vi "GUI_kHz_FlexibleDelivery.vi"() -> ()   [LabVIEW 2020]
uses:
  Shared/GUI_Template/GUI_master/tcp_new_data_event.ctl
  Shared/GUI_Template/GUI_master/tcp new data cluster.ctl
panel:
  in  "BASE PATH":path=path "Z:/software/control-all-loasis/kHzLPA/Active Version"
  in  "stop":bool=TRUE
  in  "Tab Control":T1(tab)=enum."Experts Only"
  in  "GUIdevice 19":string="kHz_Cam2-3_AstrellaMode"
  in  "GUIdevice 14":string="KHz_Cam68-1_ghost"
  in  "GUIdevice 13":string="kHz_Cam1-4_Astrella-Spol"
  in  "GUIdevice 6":string="kHz_Pico8742_EC"
  in  "GUIdevice 2":string="kHz_1Wire"
  in  "GUIdevice 1":string="kHz_ManualParameter"
  in  "GUIdevice 3":string="kHz_Zaber_Vacuum"
  in  "GUIdevice 4":string="kHz_DG645_ShotControl"
  in  "GUIdevice 5":string="kHz_Pico8742_CC"
  out "error IO":errorcluster
  out "tcp data event":T2
  in  "GUIdevice 7":string="kHz_ESP_TC"
  in  "GUIdevice 8":string="kHz_Pico8742_GLO"
  in  "GUIdevice 9":string="kHz_Pico8742_ROT"
  in  "GUIdevice 10":string="kHz_FilterWheel_splitter"
  in  "GUIdevice 11":string="kHz_Cam42-4_NFProfileOL"
  in  "GUIdevice 12":string="kHz_Cam42-2_EC"
  in  "GUIdevice 15":string="kHz_Cam42-2_EC"
  in  "GUIdevice 16":string="kHz_Cam42-4_NFProfileOL"
  in  "GUIdevice 18":string="kHz_Cam68-3_MantaG-158"
  in  "GUIdevice 17":string="kHz_Cam68-2_SpolGhost"
  in  "Position.Channel 1::2":T3(ring) caption="Mode Flipper"
  in  "step size EC":i32=200 caption="Step Size" min=10 max=1000 step=10
  in  "step size GLO":i32=200 caption="Step Size" min=10 max=1000 step=10
  in  "step size CC":i32=200 caption="Step Size" min=10 max=1000 step=10
  in  "value8::1":i8=-3 caption="Round Trip" min=-4 max=0 step=1 format="%.0g"
  in  "value7::1":dbl=35.0 caption="HWP attenuator" min=-9999999.0 max=9999999.0
  out "HCF output energy":dbl=7.782297644090318 caption="HCF output energy [uJ]"
  in  "Position.device 3::6":i32=450 caption="EC H" min=-1000 max=1000 step=200
  in  "Position.device 4::6":i32=1350 caption="EC V" min=-1000 max=1000 step=200
  in  "Position.device 1::5":i32=-8149 caption="Near H" min=-20000 max=20000 step=50
  in  "Position.device 2::5":i32=-10850 caption="Near V" min=-20000 max=20000 step=50
  in  "Position.device 1::8":i32=100 caption="Far V" min=-100000 max=100000 step=200
  in  "Position.device 2::8":i32=-69835 caption="Far H" min=-100000 max=100000 step=200
  in  "Position.device 3::8":i32=-48990 caption="OAP V" min=-100000 max=100000 step=200
  in  "Position.device 4::8":i32=12420 caption="OAP H" min=-100000 max=100000 step=200
  in  "p-pol only button":bool=TRUE caption="p-pol only"
  in  "Position.Axis 3::7":dbl=23.00005 caption="Mode Wedge Position" min=0.0 max=25.0 format="%.2f"
  in  "Position.Ch2::3":dbl=53.000052 caption="Manta Cam Position" min=0.0 max=100.0 format="%.2f"
  in  "Mode Wedge Button":bool=TRUE caption="Mode Wedge In"
  in  "UDP error message":string
  out "Attenuated  Power":dbl=11.11756806298617 caption="Attenuated Power [mW]"
  out "FF input calculated":dbl=1.5564595288180636 caption="FF input  [uJ]"
  out "FF input OL":dbl=-2.9732313575525815 caption="FF input OL s+p [mW]"
  out "chart":cluster{"energy":dbl, "energy":dbl, dbl}(graph)={"energy"=-2.9732313575525815, "energy"=-2.9732313575525815, 100.0}
  out "FF Output OL":dbl=-2.9732313575525815 caption="FF output OL  [uJ]"
  in  "value10::1":dbl=0.017 caption="FF input slope" min=-9999999.0 max=9999999.0
  in  "value12::1":dbl=52.3 caption="FF Output Divisor" min=-9999999.0 max=9999999.0
  in  "MeanCounts::16":dbl caption="NFProfileOL Mean" min=0.0 max=999999999.0 format="%.2f"
  in  "pos.Channel0::10":enum16{"1", "2", "3", "4", "5", "6"}(ring)=enum."6" caption="Filter Wheel"
  in  "value5::1":dbl caption="HWP splitter" min=-9999999.0 max=9999999.0
  in  "Astrella Power":dbl[](array[numeric])=[5470.0, 3400.0, 690.0, 135.0, 20.0] caption="Astrella Power [mW]"
  in  "value1::1":dbl=21.7 caption="Revo current" min=10.0 max=30.0
  in  "exposure::16":dbl=0.001 caption="NFProfileOL exposure" min=1e-05 max=1.0 format="%.2f"
  in  "Position.device 1::9":i32=10000 caption="WP in CC" min=-10000 max=10000 step=200
  in  "step size ROT":i32=200 caption="Step Size" min=10 max=1000 step=10
  in  "MeanCounts::12":dbl caption="EC Mean" min=0.0 max=999999999.0 format="%.2f"
  in  "exposure::12":dbl=0.001 caption="EC exposure" min=1e-05 max=10.0 format="%.2f"
  in  "Max Exposure - Ghost":dbl=0.25
  in  "Max Exposure - Astrellas":dbl=0.25
  in  "GuardBand Ghost":dbl=20.0
  in  "Guardband Astrellas":dbl=100.0
  in  "Target - Ghost":dbl=170.0
  in  "Target - Astrellas":dbl=3000.0
  in  "Exposure Step Size - Ghost":dbl=0.02
  in  "Exposure Step Size - Astrellas":dbl=0.02
  in  "exposure::13":dbl=23.00005 caption="Exposure - Astrellas" min=1e-05 max=10.0 format="%.4f"
  in  "exposure::14":dbl=23.00005 caption="Exposure - Ghost" min=1e-05 max=1.0 format="%.4f"
  in  "maxcounts::13":dbl=23.00005 caption="MaxCounts - Astrellas" min=0.0 max=999999999.0 format="%.2f"
  in  "maxcounts::14":dbl=23.00005 caption="MaxCounts - Ghost" min=0.0 max=999999999.0 format="%.2f"
  in  "On":bool caption="Auto Exposure"
  out "timer":u32
  in  "Exposure Step Size -EC":dbl=0.02
  in  "Target - EC":dbl=3000.0
  in  "Max Exposure -EC":dbl=0.5
  in  "GuardBand - EC":dbl=200.0
  in  "Exposure Step Size -NFProfile":dbl=0.02
  in  "Max Exposure - NFProfile":dbl=1.0
  in  "GuardBand - NFProfile":dbl=200.0
  in  "Target -  NFProfile":dbl=3000.0
  in  "Max Exposure - SpolGhost":dbl=0.5
  in  "Exposure Step Size - SpolGhost":dbl=0.02
  in  "GuardBand - SpolGhost":dbl=200.0
  in  "Target - SpolGhost":dbl=3000.0
  in  "Max Exposure - MantaG":dbl=0.5
  in  "Exposure Step Size - MantaG":dbl=0.02
  in  "GuardBand - MantaG":dbl=200.0
  in  "Target -  MantaG":dbl=3000.0
  in  "Target -  AstrellaM":dbl
  in  "GuardBand - AstrellaM":dbl
  in  "Exposure Step Size - AstrellaM":dbl=0.02
  in  "Max Exposure - AstrellaM":dbl=1.0
  in  "maxcounts::16":dbl=23.00005 caption="MaxCounts - NFProfile" min=0.0 max=999999999.0 format="%.2f"
  in  "exposure::16":dbl=23.00005 caption="Exposure - NFProfile" min=1e-05 max=1.0 format="%.4f"
  in  "exposure::17":dbl=23.00005 caption="Exposure - SPol" min=1e-05 max=1.0 format="%.4f"
  in  "maxcounts::17":dbl=23.00005 caption="MaxCounts - SPol" min=0.0 max=999999999.0 format="%.2f"
  in  "maxcounts::18":dbl=23.00005 caption="MaxCounts - Manta" min=0.0 max=999999999.0 format="%.2f"
  in  "exposure::18":dbl=23.00005 caption="Exposure - Manta" min=1e-05 max=1.0 format="%.4f"
  in  "exposure::19":dbl=23.00005 caption="Exposure - AstrellaM" min=1e-05 max=1.0 format="%.4f"
  in  "maxcounts::19":dbl=23.00005 caption="MaxCounts - AstrellaM" min=0.0 max=999999999.0 format="%.2f"
  in  "exposure::15":dbl=23.00005 caption="Exposure - EC" min=1e-05 max=10.0 format="%.4f"
  in  "maxcounts::15":dbl=23.00005 caption="MaxCounts - EC" min=0.0 max=999999999.0 format="%.2f"
  # "Flexible Delivery"
  # "Primary Controls"
  # "Laser Status"
  # "OL Measurement"
  # "Calculated"
  # "Alignment Near-field"
  # "EC focus tuning"
  # "Beam centering on in-flange Gentec"
  # "DON'T TOUCH"
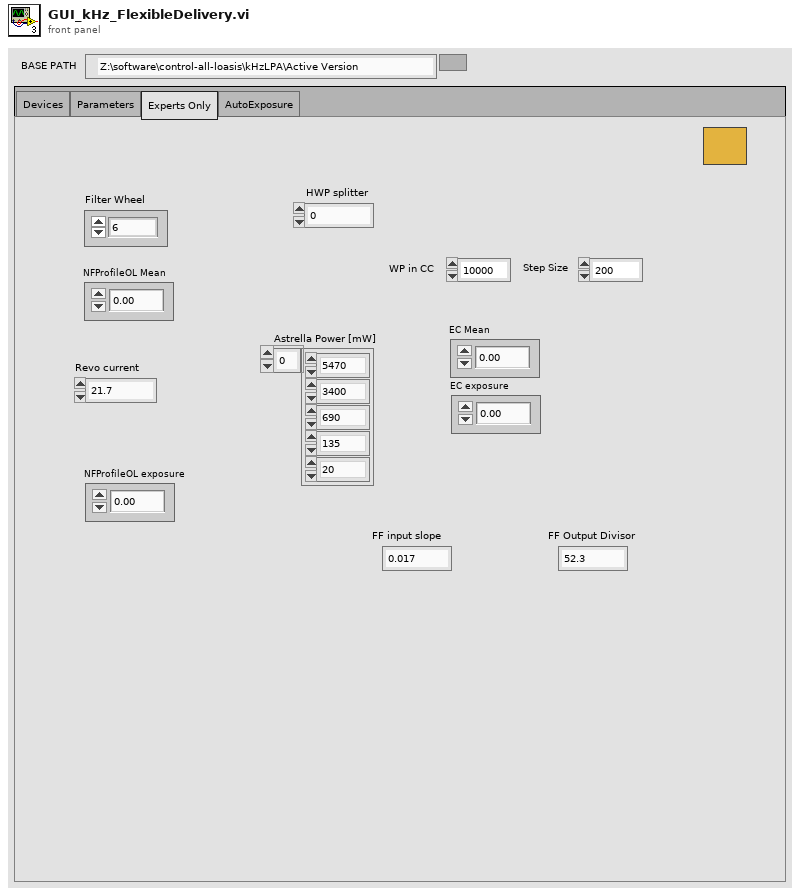
[diagram p1: front panel]
types:
  T1 = enum32{"Devices", "Parameters", "Experts Only", "AutoExposure"}
  T2 = typedef "tcp_new_data_event.ctl" = refnum<user-event>
  T3 = enum16{"Removed", "Inserted", "Unknown", "Moving"}
  T4 = typedef "tcp new data cluster.ctl" = cluster{"EventEnum":enum16{"new data", "connection status update"}, "Device name":string}
  T5 = enum32{"Invalid", "Standard", "Closed", "Hidden", "Minimized", "Maximized"}
  T6 = enum32{"invalid app kind", "Development System", "Run Time System", "Student Edition", "Embedded LabVIEW", "Evaluation", "Custom"}
  T7 = cluster{"Core":cluster{"Current VI Reference":refnum<vi>, "Close Panel on Exit?":bool}, "Tik1":u32}
  T8 = cluster{"Current VI Reference":refnum<vi>, "Close Panel on Exit?":bool}
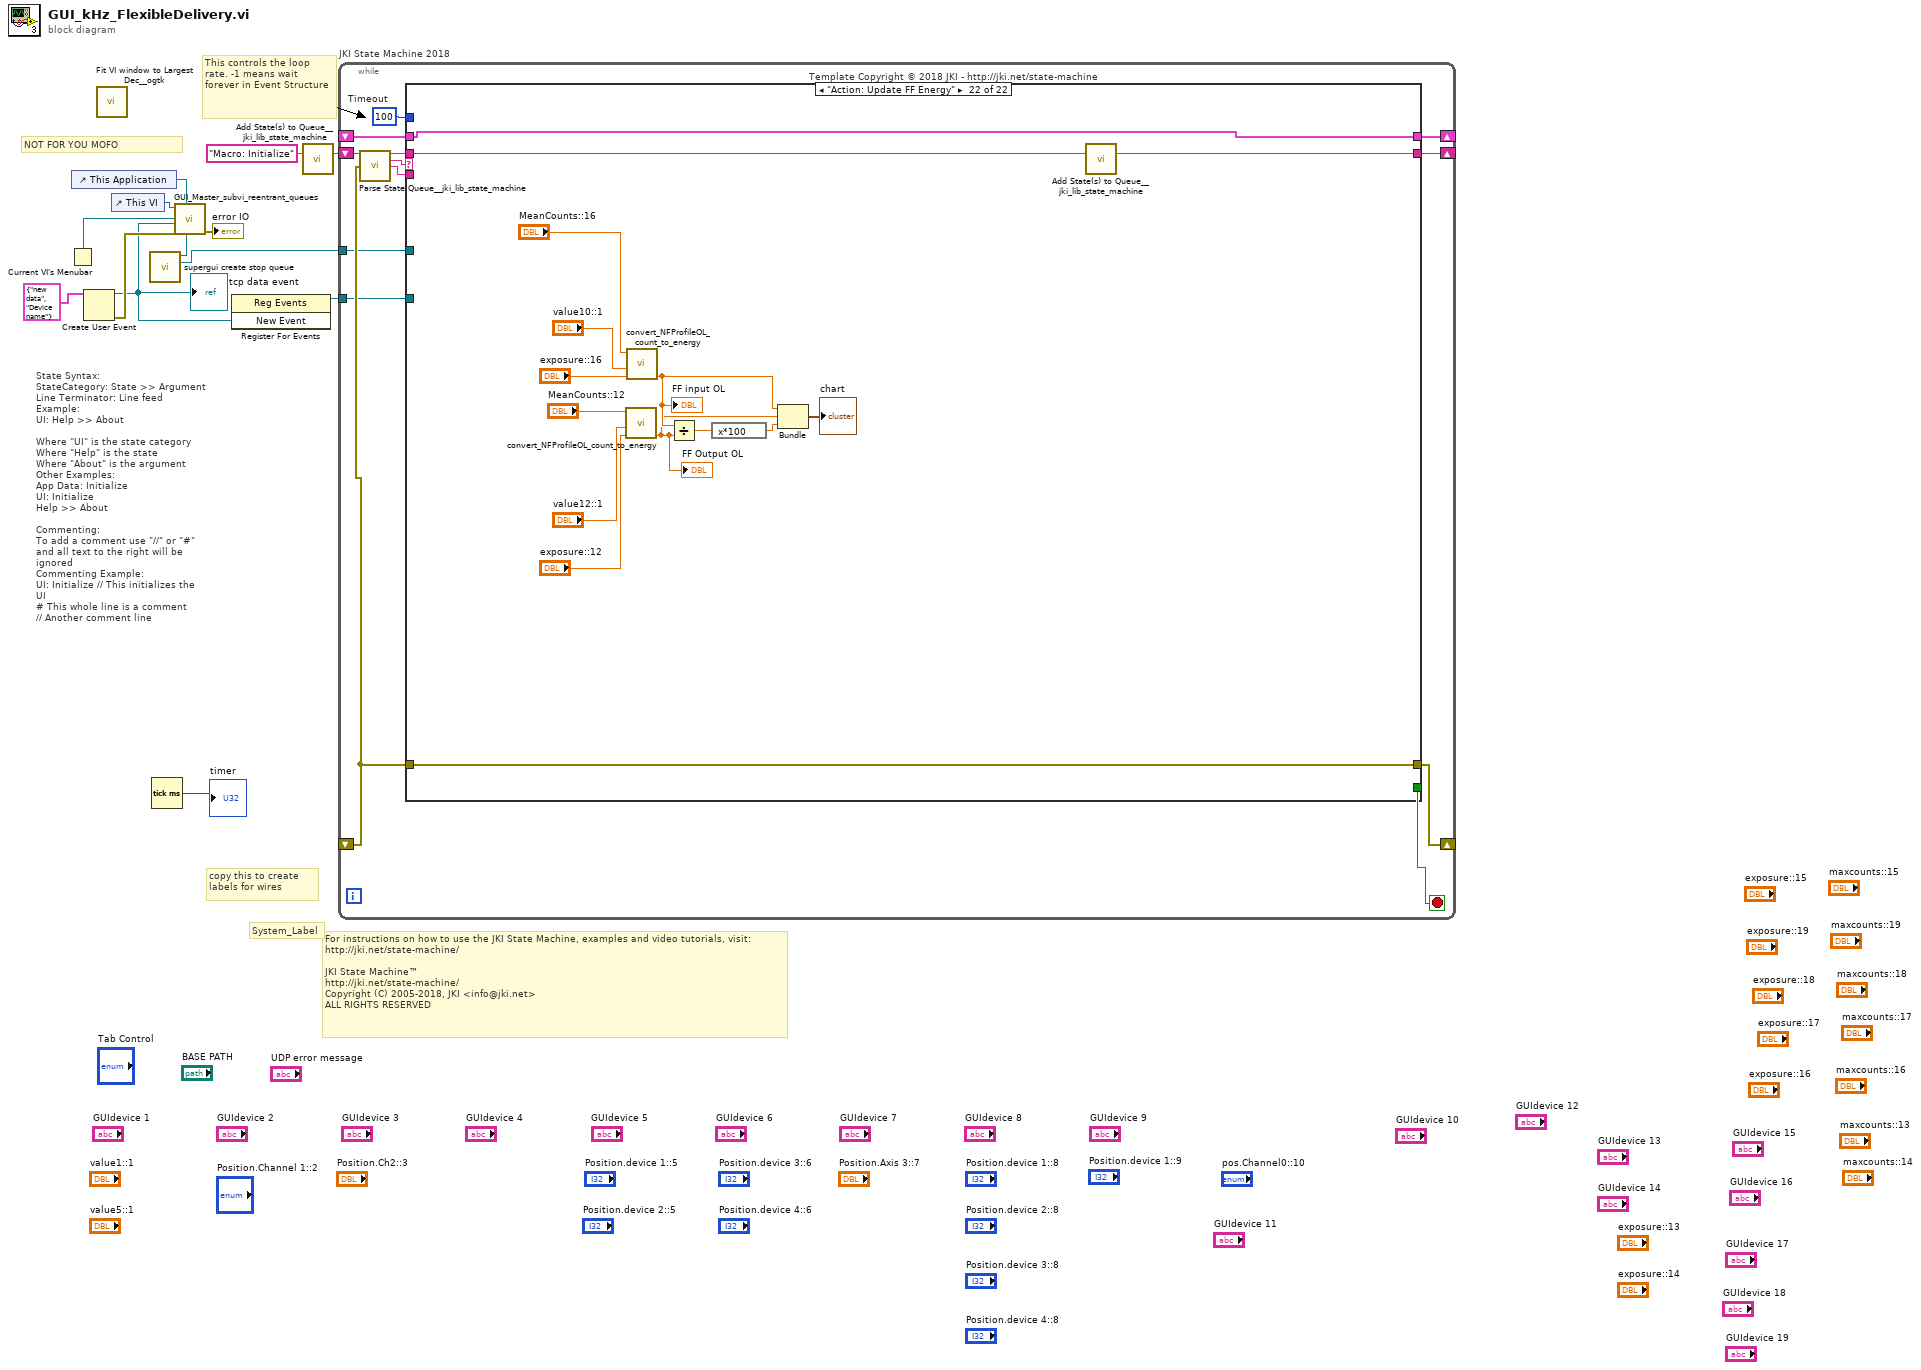
[diagram p0: block diagram]
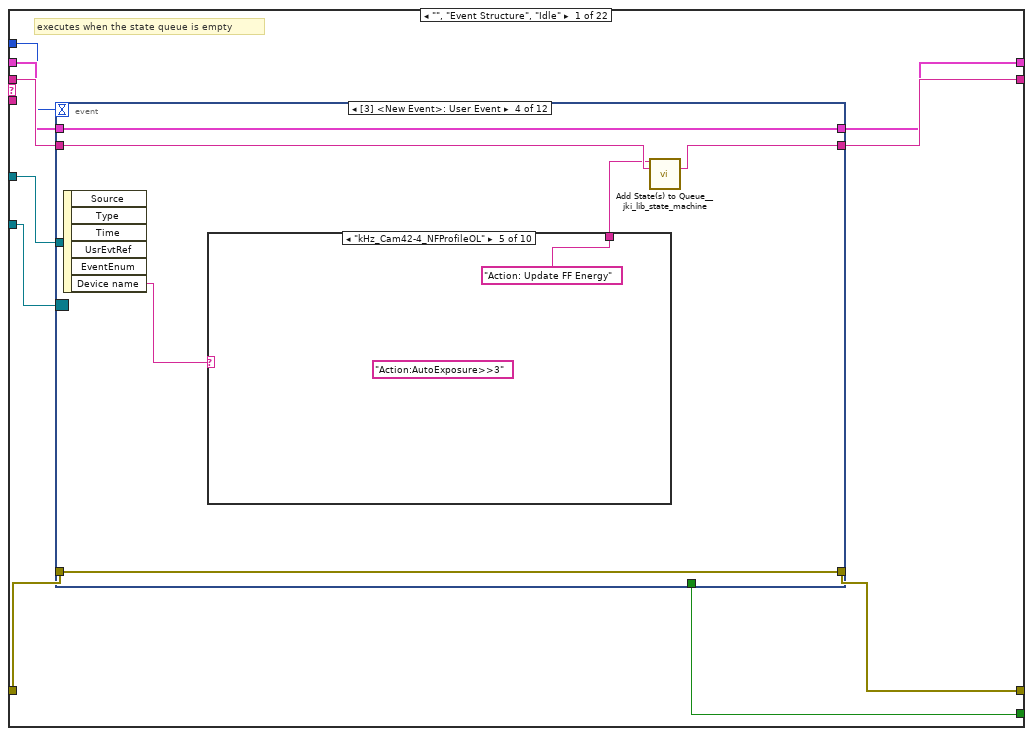
[diagram p2: hidden frame]
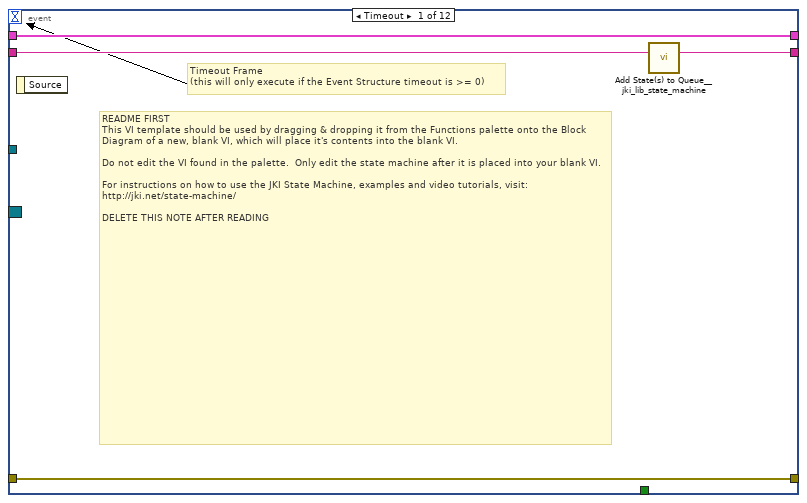
[diagram p3: hidden frame]
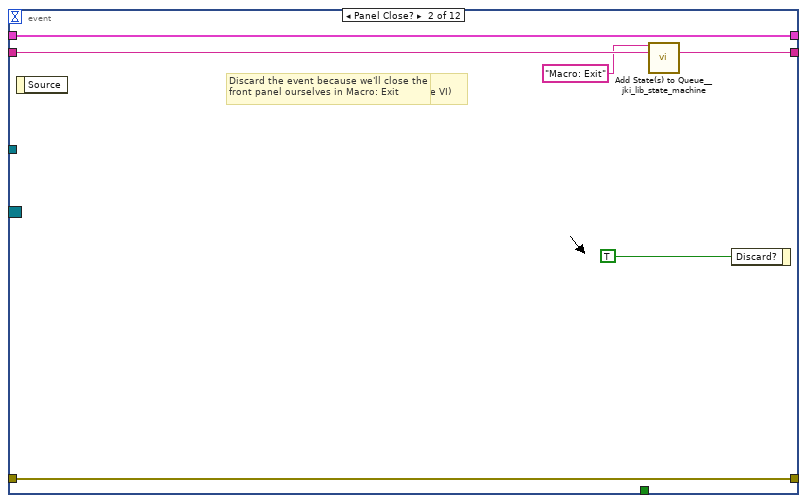
[diagram p4: hidden frame]
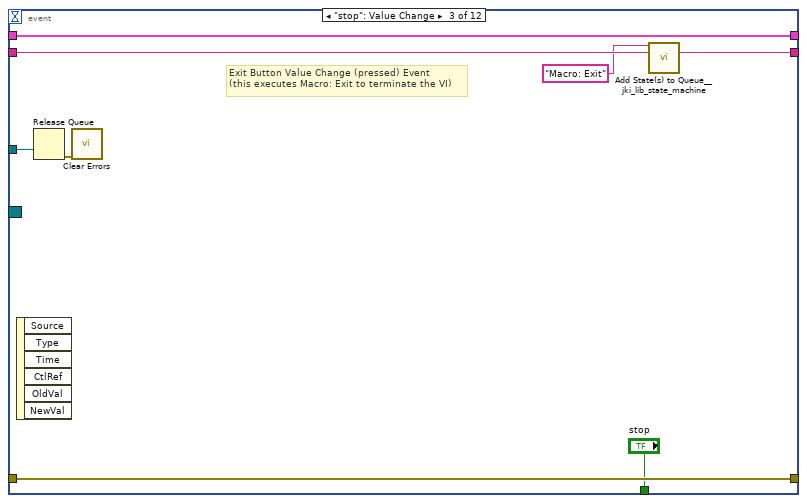
[diagram p5: hidden frame]
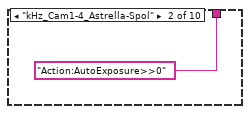
[diagram p7: hidden frame]
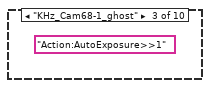
[diagram p8: hidden frame]
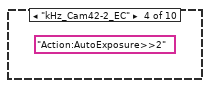
[diagram p9: hidden frame]
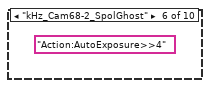
[diagram p10: hidden frame]
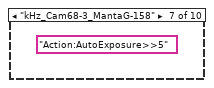
[diagram p11: hidden frame]
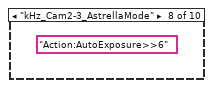
[diagram p12: hidden frame]
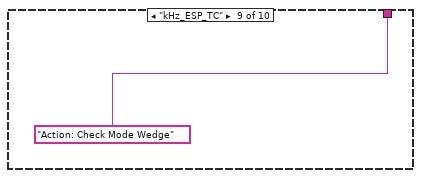
[diagram p13: hidden frame]
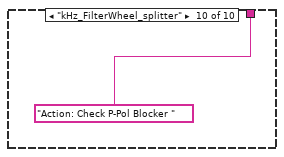
[diagram p14: hidden frame]
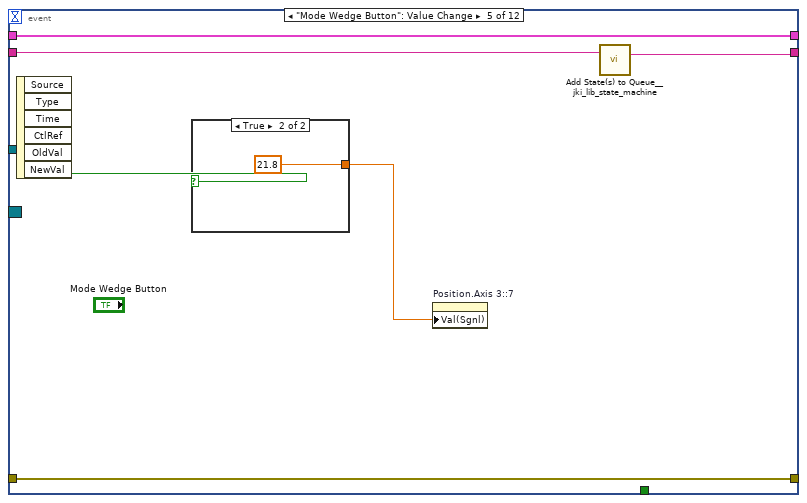
[diagram p15: hidden frame]
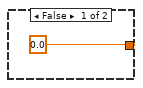
[diagram p16: hidden frame]
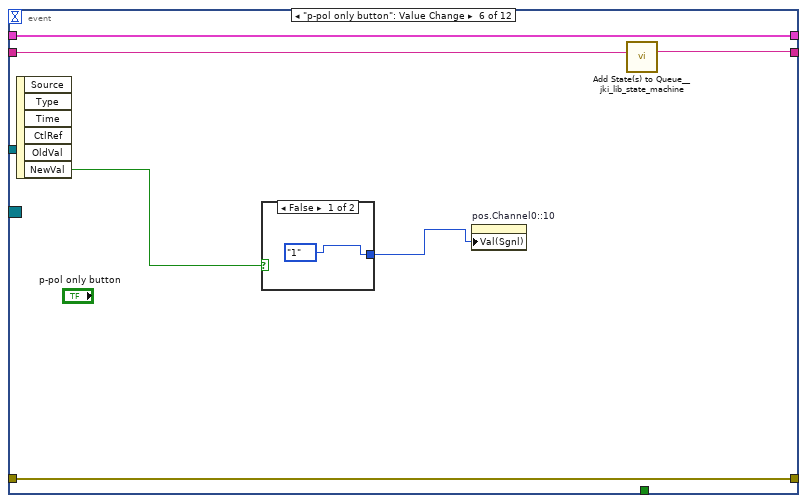
[diagram p17: hidden frame]
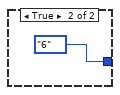
[diagram p18: hidden frame]
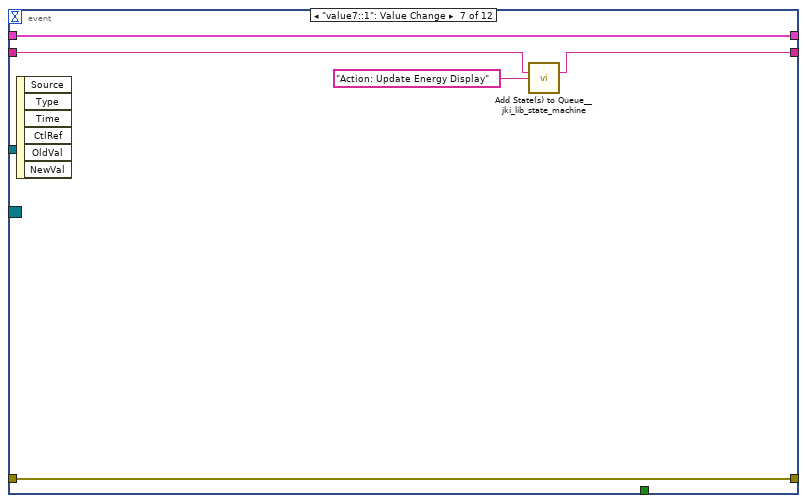
[diagram p19: hidden frame]
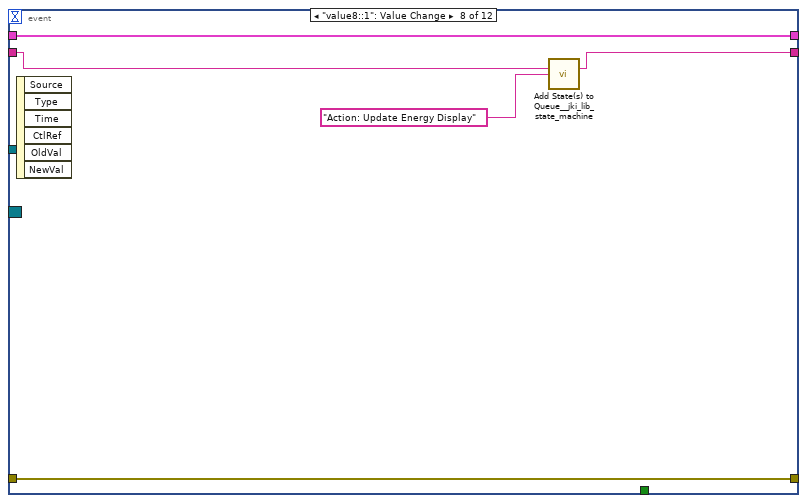
[diagram p20: hidden frame]
diagram:
  # "NOT FOR YOU MOFO"
  # "For instructions on how to use the JKI State Machine, examples and video tutorials, visit:\nhttp://jki.net/state-machine/\n\nJKI State Machine™\nhttp://jki.net/state-machine/\nCopyright (C) 2005-2018, JKI <info@jki.net>\nALL RIGHTS RESERVED"
  # "State Syntax:\nStateCategory: State >> Argument\nLine Terminator: Line feed\nExample:\nUI: Help >> About\n\nWhere \"UI\" is the state category\nWhere \"Help\" is the state\nWhere \"About\" is the argument\nOther Examples:\nApp Data: Initialize\nUI: Initialize\nHelp >> About\n\nCommenting:\nTo add a comment use \"//\" or \"#\" and all text to the right will be ignored\nCommenting Example:\nUI: Initialize // This initializes the UI\n# This whole line is a comment\n// Another comment line"
  # "copy this to create labels for wires"
  # "This controls the loop rate. -1 means wait forever in Event Structure"
  # "System_Label"
  n1 = Current VI's Menubar() -> (w7:refnum<k9>)
  n2 = control-ref of="This Application"() -> (w10:refnum<vi>)
  n3 = Create User Event(user event datatype=T4 {"EventEnum"=enum."new data", "Device name"="Device name"} ("New Event")) -> (user event=w4:refnum<user-event>, error out=w9:errorcluster)  [unwired: 1 in]
  "tcp data event" <- w4
  n4 = call <userlib>:"Fit VI window to Largest Dec__ogtk.vi"() -> ()  [unwired: 6 in, 2 out]
  n5 = control-ref of="This VI"() -> (w6:refnum<vi>)
  n6 = call "supergui create stop queue.vi"() -> ("STOP Queue out"=w3:refnum<queue>)  [unwired: 11 in]
  n7 = Tick Count (ms)() -> (millisecond timer value=→"timer":u32)
  n8 = call "GUI_Master_subvi_reentrant_queues.vi"("STOP Queue in"=w3, "This Application"=w10, "error in (no error)"=w9, "tcp data event"=w4, "Caller menu reference"=w7, "Caller VI ref"=w6) -> ("error out"=→"error IO":errorcluster)  [unwired: 5 in]
  n9 = register-events(w4) -> (reference out=w2:refnum<event-registration>)  [unwired: 2 in, 1 out]
  n10 = call <vilib>:"Add State(s) to Queue__jki_lib_state_machine.vi"("State(s) in (\"\")"="Macro: Initialize") -> ("States Out"=w12:string)  [unwired: 14 in]
  n11 = while "JKI State Machine 2018" {
    shift-right: [w18] -> _
    shift-left: _ -> [w17]
    shift-right: [w21] -> _
    shift-left: _ -> [w15]
    shift-right: [w20] -> _
    shift-left: w12 -> [w22]
    tunnel: w3 -> [w14]
    tunnel: w2 -> [w13]
    stop <- w19 stop-if-true
    w16 = 100  # Timeout
    # "Template Copyright © 2018 JKI - http://jki.net/state-machine"
    n12 = call <vilib>:"Parse State Queue__jki_lib_state_machine.vi"("State Queue"=w22, "Error In (no error)"=w15) -> ("Remaining States"=w24:string, "Current State"=w25:string, "Arguments"=w23:string)  [unwired: 11 in]
    n13 = case shown="\"Action: Update FF Energy\"" w25 {
      selector: w25 -> [_ _ w114 _ _ _ _ _ _ _ _ _ _ _ _ _ _ _ _ _ _ _]
      tunnel: w24 -> [w35 w113 w118 w137 w143 w148 w152 w159 w165 w169 w173 w179 w190 w254 w259 w269 w273 w284 w437 w444 w454 w469]
      tunnel: w23 -> [_ _ _ _ _ _ _ _ _ _ _ w174 w184 _ _ _ _ w276 _ _ _ _]
      tunnel: w17 -> [w33 w110 w116 w130 w140 w146 w149 w153 w161 w166 w171 w177 w186 w251 w256 w266 w270 w281 w429 w438 w451 w466]
      tunnel: [w32 w111 w120 w134 errorcluster {"status"=FALSE, "code"=0, "source"=""} ("error out") w145 w150 w157 w162 w167 w170 w175 w187 w252 w257 w267 w271 w282 w435 w442 w452 w467] -> w21
      tunnel: w15 -> [w31 w111 w119 w134 w139 w145 w150 w157 w163 w167 w170 w176 w188 w252 w257 w267 w271 w282 w435 w442 w452 w467]
      tunnel: [w34 w112 w117 w136 w142 w147 w151 w158 w164 w168 w172 w178 w189 w253 w258 w268 w272 w283 w436 w443 w453 w468] -> w20
      tunnel: [w27 _ _ _ _ TRUE _ _ _ _ _ _ _ _ _ _ _ _ _ _ _ _] -> w19
      tunnel: [w30 w110 w116 w135 w140 w146 w149 w154 w161 w166 w171 w177 w186 w251 w256 w266 w270 w281 w429 w438 w451 w466] -> w18
      tunnel: w16 -> [w29 _ _ _ _ _ _ _ _ _ _ _ _ _ _ _ _ _ _ _ _ _]
      tunnel: w14 -> [w28 _ _ _ _ _ _ _ _ _ _ _ _ _ _ _ _ _ _ _ _ _]
      tunnel: w13 -> [w26 _ _ _ _ _ _ _ _ _ _ _ _ _ _ _ _ _ _ _ _ _]
      frame "", "Event Structure", "Idle" {
        # "executes when the state queue is empty"
        n14 = event shown="[3] <New Event>: User Event" {
          selector: w26 -> [_ _ _ _ _ _ _ _ _ _ _ _]
          dyn-events: _ -> [_ _ _ _ _ _ _ _ _ _ _ _]
          timeout: w29 -> [_ _ _ _ _ _ _ _ _ _ _ _]
          tunnel: w35 -> [w39 w45 w53 w57 w68 w74 w84 w87 w94 w99 w104 w109]
          tunnel: [w38 w44 w52 w58 w69 w75 w83 w89 w93 w98 w103 w108] -> w34
          tunnel: w33 -> [w36 w42 w50 w59 w64 w72 w82 w88 w92 w97 w102 w107]
          tunnel: [w37 w43 w51 w54 w66 w76 w81 w86 w91 w96 w101 w106] -> w32
          tunnel: w31 -> [w37 w43 w51 w54 w66 w76 w81 w86 w91 w96 w101 w106]
          tunnel: [w36 w42 w50 w59 w64 w72 w82 w88 w92 w97 w102 w107] -> w30
          tunnel: w28 -> [_ _ w47 _ _ _ _ _ _ _ _ _]
          tunnel: [_ _ "stop" _ _ _ _ _ _ _ _ _] -> w27
          event Timeout {
            # "README FIRST\nThis VI template should be used by dragging & dropping it from the Functions palette onto the Block Diagram of a new, blank VI, which will place it's contents into the blank VI.\n\nDo not edit the VI found in the palette.  Only edit the state machine after it is placed into your blank VI.\n\nFor instructions on how to use the JKI State Machine, examples and video tutorials, visit:\nhttp://jki.net/state-machine/\n\nDELETE THIS NOTE AFTER READING"
            # "Timeout Frame\n(this will only execute if the Event Structure timeout is >= 0)"
            n15 = event-data() -> ()  [unwired: 1 in, 1 out]
            n16 = call <vilib>:"Add State(s) to Queue__jki_lib_state_machine.vi"("State(s) in (\"\")"=w39) -> ("States Out"=w38:string)  [unwired: 14 in]
          }
          event Panel Close? {
            # "Discard the event because we'll close the front panel ourselves in Macro: Exit"
            # "Close Panel button (pressed) Event\n(this executes Macro: Exit to terminate the VI)"
            n17 = event-data() -> ()  [unwired: 1 in, 1 out]
            n18 = call <vilib>:"Add State(s) to Queue__jki_lib_state_machine.vi"("State(s) in Front (\"\")"="Macro: Exit", "State(s) in (\"\")"=w45) -> ("States Out"=w44:string)  [unwired: 13 in]
            n19 = event-data("Discard?"=TRUE) -> ()  [unwired: 1 in, 1 out]
          }
          event "stop": Value Change {
            # "Exit Button Value Change (pressed) Event\n(this executes Macro: Exit to terminate the VI)"
            n20 = event-data() -> ()  [unwired: 1 in, 6 out]
            n21 = Release Queue(queue=w47) -> (error out=w48:errorcluster)  [unwired: 2 in, 2 out]
            n22 = call <vilib>:"Clear Errors.vi"("error in (no error)"=w48) -> ()  [unwired: 5 in, 2 out]
            n23 = call <vilib>:"Add State(s) to Queue__jki_lib_state_machine.vi"("State(s) in Front (\"\")"="Macro: Exit", "State(s) in (\"\")"=w53) -> ("States Out"=w52:string)  [unwired: 13 in]
          }
          event User Event {
            n24 = event-data() -> ("Device name"=w56:string)  [unwired: 1 in, 5 out]
            n25 = case shown="\"kHz_Cam42-4_NFProfileOL\"" w56 {
              tunnel: [_ "Action:AutoExposure>>0" _ _ "Action: Update FF Energy" ("State(s) in Front (\"\")") _ _ _ "Action: Check Mode Wedge" ("State(s) in Front (\"\")") "Action: Check P-Pol Blocker " ("State(s) in Front (\"\")")] -> w55
              frame "False", Default {
              }
              frame "kHz_Cam1-4_Astrella-Spol" {
              }
              frame "KHz_Cam68-1_ghost" {
                (unwired) "Action:AutoExposure>>1"
              }
              frame "kHz_Cam42-2_EC" {
                (unwired) "Action:AutoExposure>>2"
              }
              frame "kHz_Cam42-4_NFProfileOL" {
                (unwired) "Action:AutoExposure>>3"
              }
              frame "kHz_Cam68-2_SpolGhost" {
                (unwired) "Action:AutoExposure>>4"
              }
              frame "kHz_Cam68-3_MantaG-158" {
                (unwired) "Action:AutoExposure>>5"
              }
              frame "kHz_Cam2-3_AstrellaMode" {
                (unwired) "Action:AutoExposure>>6"
              }
              frame "kHz_ESP_TC" {
              }
              frame "kHz_FilterWheel_splitter" {
              }
            }
            n26 = call <vilib>:"Add State(s) to Queue__jki_lib_state_machine.vi"("State(s) in Front (\"\")"=w55, "State(s) in (\"\")"=w57) -> ("States Out"=w58:string)  [unwired: 13 in]
          }
          event "Mode Wedge Button": Value Change {
            n27 = event-data() -> ("NewVal"=w67:bool)  [unwired: 1 in, 5 out]
            n28 = case shown="True" w67 {
              tunnel: [0.0 ("opening Time") 21.8] -> w65
              frame False {
              }
              frame True {
              }
            }
            n29 = property on="Position.Axis 3::7" class="DigNum (strict)"("Val(Sgnl)"=w65) -> ()  [unwired: 2 in, 2 out]
            n30 = call <vilib>:"Add State(s) to Queue__jki_lib_state_machine.vi"("State(s) in (\"\")"=w68) -> ("States Out"=w69:string)  [unwired: 14 in]
          }
          event "p-pol only button": Value Change {
            n31 = event-data() -> ("NewVal"=w77:bool)  [unwired: 1 in, 5 out]
            n32 = case shown="False" w77 {
              tunnel: [enum16{"1", "2", "3", "4", "5", "6"}."1" ("pos.Channel0::10") enum16{"1", "2", "3", "4", "5", "6"}."6" ("pos.Channel0::10")] -> w73
              frame False {
              }
              frame True {
              }
            }
            n33 = property on="pos.Channel0::10" class="Enum (strict)"("Val(Sgnl)"=w73) -> ()  [unwired: 2 in, 2 out]
            n34 = call <vilib>:"Add State(s) to Queue__jki_lib_state_machine.vi"("State(s) in (\"\")"=w74) -> ("States Out"=w75:string)  [unwired: 14 in]
          }
          event "value7::1": Value Change {
            n35 = event-data() -> ()  [unwired: 1 in, 6 out]
            n36 = call <vilib>:"Add State(s) to Queue__jki_lib_state_machine.vi"("State(s) in (\"\")"=w84, "State(s) at Back (\"\")"="Action: Update Energy Display" ("State(s) at Back (\"\")")) -> ("States Out"=w83:string)  [unwired: 13 in]
          }
          event "value8::1": Value Change {
            n37 = event-data() -> ()  [unwired: 1 in, 6 out]
            n38 = call <vilib>:"Add State(s) to Queue__jki_lib_state_machine.vi"("State(s) in (\"\")"=w87, "State(s) at Back (\"\")"="Action: Update Energy Display" ("State(s) at Back (\"\")")) -> ("States Out"=w89:string)  [unwired: 13 in]
          }
          event "step size CC": Value Change {
            n39 = event-data() -> ("NewVal"=w90:i32)  [unwired: 1 in, 5 out]
            n40 = property on="Position.device 1::5" class="DigNum (strict)"("Increment"=w90) -> ()  [unwired: 2 in, 2 out]
            n41 = property on="Position.device 2::5" class="DigNum (strict)"("Increment"=w90) -> ()  [unwired: 2 in, 2 out]
            n42 = call <vilib>:"Add State(s) to Queue__jki_lib_state_machine.vi"("State(s) in (\"\")"=w94) -> ("States Out"=w93:string)  [unwired: 14 in]
          }
          event "step size EC": Value Change {
            n43 = event-data() -> ("NewVal"=w95:i32)  [unwired: 1 in, 5 out]
            n44 = property on="Position.device 3::6" class="DigNum (strict)"("Increment"=w95) -> ()  [unwired: 2 in, 2 out]
            n45 = property on="Position.device 4::6" class="DigNum (strict)"("Increment"=w95) -> ()  [unwired: 2 in, 2 out]
            n46 = call <vilib>:"Add State(s) to Queue__jki_lib_state_machine.vi"("State(s) in (\"\")"=w99) -> ("States Out"=w98:string)  [unwired: 14 in]
          }
          event "step size GLO": Value Change {
            n47 = event-data() -> ("NewVal"=w100:i32)  [unwired: 1 in, 5 out]
            n48 = property on="Position.device 1::8" class="DigNum (strict)"("Increment"=w100) -> ()  [unwired: 2 in, 2 out]
            n49 = property on="Position.device 2::8" class="DigNum (strict)"("Increment"=w100) -> ()  [unwired: 2 in, 2 out]
            n50 = property on="Position.device 3::8" class="DigNum (strict)"("Increment"=w100) -> ()  [unwired: 2 in, 2 out]
            n51 = property on="Position.device 4::8" class="DigNum (strict)"("Increment"=w100) -> ()  [unwired: 2 in, 2 out]
            n52 = call <vilib>:"Add State(s) to Queue__jki_lib_state_machine.vi"("State(s) in (\"\")"=w104) -> ("States Out"=w103:string)  [unwired: 14 in]
          }
          event "step size ROT": Value Change {
            n53 = event-data() -> ("NewVal"=w105:i32)  [unwired: 1 in, 5 out]
            n54 = property on="Position.device 1::9" class="DigNum (strict)"("Increment"=w105) -> ()  [unwired: 2 in, 2 out]
            n55 = call <vilib>:"Add State(s) to Queue__jki_lib_state_machine.vi"("State(s) in (\"\")"=w109) -> ("States Out"=w108:string)  [unwired: 14 in]
          }
        }
      }
      frame "---------- Core ----------" {
        # "Do not put any code in this frame.\n(it is a separator no-op)"
        n56 = call <vilib>:"Add State(s) to Queue__jki_lib_state_machine.vi"("State(s) in (\"\")"=w113) -> ("States Out"=w112:string)  [unwired: 14 in]
      }
      frame Default {
        w123 = 42 items=["No error", "Argument error", "Memory is full", "Out of zone", "End of file", "File already open", "Generic file I/O error", "File not found", "File permission error", "Disk is full", "Duplicate path", "Too many files open", "System feature not enabled", "Resource file not found", "Cannot add resource", "Resource not found", "Image not found", "Image memory error", "Pen does not exist", "Config type invalid", "Config token not found", "Config parse error", "Config memory error", "Bad external code format", "Bad external code offset", "External code not present", "Null window", "Destroy window error", "Null menu", "Print aborted", "Bad print record", "Print driver error", "Windows error during printing", "Memory error during printing", "Print dialog error", "Generic print error", "Invalid device refnum", "Device not found", "Device parameter error", "Device unit error", "Cannot open device", "Device call aborted", "Generic error", "Cancelled by user", "Object ID too low", "Object ID too high", "Object not in heap", "Unknown heap", "Unknown object (invalid DefProc)", "Unknown object (DefProc not in table)", "Message out of range", "Invalid (null) method", "Unknown message", "Manager call not supported", "Bad address", "Network operation in progress", "Network operation timed out", "Connection is busy", "Network attribute not supported", "Network error", "Address in use", "System out of memory", "Connection aborted", "Connection refused", "Not connected", "Already connected", "Connection closed", "Initialization error (interapplication manager)", "Bad occurrence", "Wait on unbound occurrence handler", "Occurrence queue overflow", "Datalog type conflict", "Unused", "Unrecognized type (interapplication manager)", "Memory corrupt", "Failed to make temporary DLL", "Old CIN version", "Drag socket not found", "Failed to load drop-object", "Failed to register OLE object", "Failed to release OLE object", "Format specifier type mismatch", "Unknown format specifier", "Too few format specifiers", "Too many format specifiers", "Scan failed", "Newer CIN version", "Error converting to variant", "Runtime menu error", "Password tampered", "Variant attribute not found", "Incompatible variant data type", "Event data is not available", "Event Store is not present", "Occurrence is not found", "Event Queue is not created", "Event info is not available", "Refnum passed is NULL", "Error retrieving Class GUID", "Error retrieving CoClass GUID", "Error retrieving TypeLib GUID.", "Bad built application magic bytes.", "Specific driver is different from the specific driver associated with the Logical Name.", "There is no session opened to the class driver.", "Max Error", "MAX - Error with config objects", "MAX - Error loading configuration", "MAX - Group not supported"]
        # "Current State"
        # "Do not delete, rename, or modify this frame.\n(this is used to capture unhandled states and typos)"
        # "Handle mistyped state name (developer tool)"
        n57 = Format Into String(format string="Software Exception: Unhandled State \"%s\"." ("message"), error in=w119, w114) -> (resulting string=w122:string, error out=w121:errorcluster)  [unwired: 1 in]
        n58 = call <vilib>:"Error Cluster From Error Code.vi"("show call chain? (False)"=TRUE, "error in (no error)"=w121, "error message (\"\")"=w122, "error code (0)"=w123) -> ("error out"=w120:errorcluster)  [unwired: 5 in]
        n59 = call <vilib>:"Add State(s) to Queue__jki_lib_state_machine.vi"("State(s) in (\"\")"=w118) -> ("States Out"=w117:string)  [unwired: 14 in]
      }
      frame "Initialize Core Data" {
        # "Do not delete, rename, or modify this frame.\n(this is used to determine panel behavior on exit)"
        # "originally closed?"
        # "exe?"
        # "If panel starts closed or is an EXE, then close it when we exit"
        n60 = property class="VI"() -> ("FP.State"=w127:T5)  [unwired: 2 in, 2 out]
        n61 = property class="App"() -> ("App.Kind"=w133:T6)  [unwired: 2 in, 2 out]
        n62 = control-ref of="Current VI Reference"() -> (w128:refnum<vi>)
        n63 = Equal?(x=w127, y=T5."Closed" ("Front Panel Window:State")) -> (x = y?=w125:bool)
        n64 = Equal?(x=w133, y=T6."Run Time System" ("Application:Kind")) -> (x = y?=w131:bool)
        n65 = Or(x=w125, y=w131) -> (x .or. y?=w129:bool)
        n66 = Bundle By Name(cluster=w130, "Core.Current VI Reference"=w128, "Core.Close Panel on Exit?"=w129) -> (w135:T7)
        n67 = call <vilib>:"Add State(s) to Queue__jki_lib_state_machine.vi"("State(s) in (\"\")"=w137) -> ("States Out"=w136:string)  [unwired: 14 in]
      }
      frame "Error Handler" {
        # "Unhandled Error -- Display it"
        # "Handle any errors here.\nYou can also output any states to clean-up after errors occur"
        # "Clear error"
        n68 = call <vilib>:"General Error Handler.vi"("error in (no error)"=w139) -> ()  [unwired: 10 in, 5 out]
        n69 = call <vilib>:"Add State(s) to Queue__jki_lib_state_machine.vi"("State(s) in Front (\"\")"="/* Post Error States", "State(s) in (\"\")"=w143) -> ("States Out"=w142:string)  [unwired: 13 in]
      }
      frame "Exit" {
        # "Do not put any code in this frame.\n(No errors that occur here will be handled.)"
        n70 = call <vilib>:"Add State(s) to Queue__jki_lib_state_machine.vi"("State(s) in (\"\")"=w148) -> ("States Out"=w147:string)  [unwired: 14 in]
      }
      frame "---------- Data ----------" {
        # "Do not put any code in this frame.\n(It is a separator no-op. You can make a copy of this frame to create a new Data frame)"
        n71 = call <vilib>:"Add State(s) to Queue__jki_lib_state_machine.vi"("State(s) in (\"\")"=w152) -> ("States Out"=w151:string)  [unwired: 14 in]
      }
      frame "Data: Initialize" {
        w155 = u32 0  # Tik1
        w156 = T8 {"Current VI Reference"=refnum, "Close Panel on Exit?"=FALSE}  # Core
        # "do not delete - used by framework"
        # "Expand Bundle to add new data elements to shift register data."
        # "Add new data here."
        # "Data names and types of shift register data are defined by this bundle."
        # "Initialize the shift-register data, here.\n(data names are defined by what you wire into the bundle function)"
        n72 = Bundle(cluster=w153, "Core"=w156, "Tik1"=w155) -> (w154:T7)
        n73 = call <vilib>:"Add State(s) to Queue__jki_lib_state_machine.vi"("State(s) in (\"\")"=w159) -> ("States Out"=w158:string)  [unwired: 14 in]
      }
      frame "Data: Cleanup" {
        # "Cleanup any data and references, here.\n(this is called automatically, by the Macro: Exit)"
        n74 = Unbundle By Name(w161) -> ("Core.Current VI Reference"=w160:refnum<vi>)
        n75 = Close Reference(reference=w160, error in (no error)=w163) -> (error out=w162:errorcluster)
        n76 = call <vilib>:"Add State(s) to Queue__jki_lib_state_machine.vi"("State(s) in (\"\")"=w165) -> ("States Out"=w164:string)  [unwired: 14 in]
      }
      frame "---------- UI ----------" {
        # "Do not put any code in this frame.\n(It is a separator no-op. You can make a copy of this frame to create a new UI frame)"
        n77 = call <vilib>:"Add State(s) to Queue__jki_lib_state_machine.vi"("State(s) in (\"\")"=w169) -> ("States Out"=w168:string)  [unwired: 14 in]
      }
      frame "UI: Initialize" {
        # "Initialize the User Interface, here.\n(this is called automatically, by the Macro: Init)"
        n78 = call <vilib>:"Add State(s) to Queue__jki_lib_state_machine.vi"("State(s) in (\"\")"=w173) -> ("States Out"=w172:string)  [unwired: 14 in]
      }
      frame "UI: Cursor Set" {
        # "Argument"
        # "Set and Unset Cursor Busy.\n(Usage: \"UI: Cursor Set >> Busy|Idle\")"
        n79 = case shown="\"Idle\", Default" w174 {
          tunnel: w176 -> [w181 w183]
          tunnel: [w180 w182] -> w175
          frame "Idle", Default {
            n80 = call <vilib>:"Unset Busy.vi"("error in (no error)"=w181) -> ("error out"=w180:errorcluster)  [unwired: 10 in]
          }
          frame "Busy" {
            n81 = call <vilib>:"Set Busy.vi"("error in (no error)"=w183) -> ("error out"=w182:errorcluster)  [unwired: 9 in, 1 out]
          }
        }
        n82 = call <vilib>:"Add State(s) to Queue__jki_lib_state_machine.vi"("State(s) in (\"\")"=w179) -> ("States Out"=w178:string)  [unwired: 14 in]
      }
      frame "UI: Front Panel State" {
        # "Argument"
        # "Set Front Panel Open or Closed\n(Usage: \"UI: Front Panel State >> Open|Close\")"
        n83 = Unbundle By Name(w186) -> ("Core.Current VI Reference"=w185:refnum<vi>)
        n84 = case shown="\"Close\", \"Closed\"" w184 {
          tunnel: w188 -> [w196 w209 w220 w232 w244]
          tunnel: [w197 w210 w221 w233 w245] -> w187
          tunnel: w185 -> [_ _ _ _ _]
          frame "Open", "Standard", Default {
            w191 = T5."Standard" ("State")
            n85 = property class="VI"(error in=w196) -> (reference out=w194:refnum<vi>, error out=w195:errorcluster, "FP.State"=w193:T5)  [unwired: 1 in]
            n86 = Not Equal?(x=w193, y=w191) -> (x != y?=w192:bool)
            n87 = case shown="True" w192 {
              tunnel: [w201 w203] -> w197
              tunnel: w195 -> [w200 w203]
              tunnel: w194 -> [w199 _]
              tunnel: w191 -> [w198 _]
              frame True {
                n88 = invoke class="VI" method="FP.Open"(reference=w199, error in=w200, "Activate"=TRUE, "State"=w198) -> (error out=w201:errorcluster)  [unwired: 1 in, 4 out]
              }
              frame False {
              }
            }
          }
          frame "Close", "Closed" {
            n89 = property class="VI"(error in=w209) -> (reference out=w207:refnum<vi>, error out=w208:errorcluster, "FP.State"=w205:T5)  [unwired: 1 in]
            n90 = Not Equal?(x=w205, y=T5."Closed" ("Front Panel Window:State")) -> (x != y?=w204:bool)
            n91 = case shown="True" w204 {
              tunnel: [w211 w214] -> w210
              tunnel: w208 -> [w211 w213]
              tunnel: w207 -> [_ w212]
              frame False {
              }
              frame True {
                n92 = invoke class="VI" method="FP.Close"(reference=w212, error in=w213) -> (error out=w214:errorcluster)  [unwired: 1 in, 2 out]
              }
            }
          }
          frame "Hidden", "Hide" {
            w215 = T5."Hidden" ("State")
            n93 = property class="VI"(error in=w220) -> (reference out=w218:refnum<vi>, error out=w219:errorcluster, "FP.State"=w217:T5)  [unwired: 1 in]
            n94 = Not Equal?(x=w217, y=w215) -> (x != y?=w216:bool)
            n95 = case shown="True" w216 {
              tunnel: [w225 w226] -> w221
              tunnel: w219 -> [w224 w226]
              tunnel: w218 -> [w223 _]
              tunnel: w215 -> [w222 _]
              frame True {
                n96 = invoke class="VI" method="FP.Open"(reference=w223, error in=w224, "State"=w222) -> (error out=w225:errorcluster)  [unwired: 2 in, 4 out]
              }
              frame False {
              }
            }
          }
          frame "Minimize", "Minimized" {
            w227 = T5."Minimized" ("State")
            n97 = property class="VI"(error in=w232) -> (reference out=w230:refnum<vi>, error out=w231:errorcluster, "FP.State"=w229:T5)  [unwired: 1 in]
            n98 = Not Equal?(x=w229, y=w227) -> (x != y?=w228:bool)
            n99 = case shown="True" w228 {
              tunnel: [w237 w238] -> w233
              tunnel: w231 -> [w236 w238]
              tunnel: w230 -> [w235 _]
              tunnel: w227 -> [w234 _]
              frame True {
                n100 = invoke class="VI" method="FP.Open"(reference=w235, error in=w236, "State"=w234) -> (error out=w237:errorcluster)  [unwired: 2 in, 4 out]
              }
              frame False {
              }
            }
          }
          frame "Maximize", "Maximized" {
            w239 = T5."Maximized" ("State")
            n101 = property class="VI"(error in=w244) -> (reference out=w242:refnum<vi>, error out=w243:errorcluster, "FP.State"=w241:T5)  [unwired: 1 in]
            n102 = Not Equal?(x=w241, y=w239) -> (x != y?=w240:bool)
            n103 = case shown="True" w240 {
              tunnel: [w249 w250] -> w245
              tunnel: w243 -> [w248 w250]
              tunnel: w242 -> [w247 _]
              tunnel: w239 -> [w246 _]
              frame True {
                n104 = invoke class="VI" method="FP.Open"(reference=w247, error in=w248, "State"=w246) -> (error out=w249:errorcluster)  [unwired: 2 in, 4 out]
              }
              frame False {
              }
            }
          }
        }
        n105 = call <vilib>:"Add State(s) to Queue__jki_lib_state_machine.vi"("State(s) in (\"\")"=w190) -> ("States Out"=w189:string)  [unwired: 14 in]
      }
      frame "---------- Macro ----------" {
        # "Do not put any code in this frame.\n(It is a separator no-op. You can make a copy of this frame to create a new Macro frame)"
        n106 = call <vilib>:"Add State(s) to Queue__jki_lib_state_machine.vi"("State(s) in (\"\")"=w254) -> ("States Out"=w253:string)  [unwired: 14 in]
      }
      frame "Macro: Initialize" {
        w255 = "Data: Initialize\nInitialize Core Data\nAction: Check Mode Wedge\nAction: Check P-Pol Blocker\nAction: Update Energy Display\nUI: Initialize\nUI: Front Panel State >> Open"  # Data: Initialize Initialize Core Data Action: Check Mode Wedge Action: Check P-Pol Blocker Action: Update Energy Display UI: Initialize UI: Front Panel State >> Open
        # "Initialization Macro\n(This is called once, when the VI starts)"
        n107 = call <vilib>:"Add State(s) to Queue__jki_lib_state_machine.vi"("State(s) in Front (\"\")"=w255, "State(s) in (\"\")"=w259) -> ("States Out"=w258:string)  [unwired: 13 in]
      }
      frame "Macro: Exit" {
        # "Exit Macro\n(This is called once, when the VI exits)"
        n108 = Unbundle By Name(w266) -> ("Core.Close Panel on Exit?"=w260:bool)
        n109 = Select(t="UI: Front Panel State >> Close", s=w260, f="") -> (s? t:f=w263:string)
        n110 = call <vilib>:"Add State(s) to Queue__jki_lib_state_machine.vi"("State(s) in (\"\")"=w263, "State(s) at Back (\"\")"="Data: Cleanup\nExit") -> ("States Out"=w261:string)  [unwired: 13 in]
        n111 = call <vilib>:"Add State(s) to Queue__jki_lib_state_machine.vi"("State(s) in Front (\"\")"=w261, "State(s) in (\"\")"=w269) -> ("States Out"=w268:string)  [unwired: 13 in]
      }
      frame "---------- Action ----------" {
        # "Template Separator\n(You can make a copy of, or modify, this frame)"
        n112 = call <vilib>:"Add State(s) to Queue__jki_lib_state_machine.vi"("State(s) in (\"\")"=w273) -> ("States Out"=w272:string)  [unwired: 14 in]
      }
      frame "Action:AutoExposure" {
        # "Template Separator\n(You can make a copy of, or modify, this frame)"
        n113 = local read "timer"() -> (w279:u32)
        n114 = Tick Count (ms)() -> (millisecond timer value=w280:u32)
        n115 = Decimal String To Number(string=w276) -> (number=w275:i32)  [unwired: 2 in, 1 out]
        n116 = Subtract(x=w280, y=w279) -> (x-y=w278:u32)
        n117 = Greater?(x=w278, y=u32 750) -> (0:w274:bool)
        n118 = case shown="True" w274 {
          tunnel: w275 -> [_ w285]
          frame False {
          }
          frame True {
            n119 = Tick Count (ms)() -> (millisecond timer value=w286:u32)
            n120 = case shown="True" "On" {
              tunnel: w285 -> [_ _]
              frame False {
              }
              frame True {
                n121 = stacked-sequence {
                  frame #0 {
                    n122 = property on="maxcounts::13" class="DigNum (strict)"() -> ("Value"=w290:dbl)  [unwired: 2 in, 2 out]
                    n123 = Subtract(x="Target - Astrellas", y=w290) -> (x-y=w288:dbl)
                    n124 = Absolute Value(x=w288) -> (abs(x)=w293:dbl)
                    n125 = Greater?(x=w293, y="Guardband Astrellas") -> (0:w291:bool)
                    n126 = case shown="True" w291 {
                      tunnel: w288 -> [_ w300]
                      frame False {
                      }
                      frame True {
                        n127 = Greater Than 0?(x=w300) -> (x > 0?=w299:bool)
                        n128 = property on="exposure::13" class="DigNum (strict)"() -> ("Value"=w298:dbl)  [unwired: 2 in, 2 out]
                        n129 = case shown="True" w299 {
                          tunnel: w298 -> [w302 w306]
                          tunnel: "Exposure Step Size - Astrellas" -> [w303 w307]
                          tunnel: [w304 w305] -> w296
                          frame False {
                            n130 = Subtract(x=w302, y=w303) -> (x-y=w304:dbl)
                          }
                          frame True {
                            n131 = Add(x=w306, y=w307) -> (x+y=w305:dbl)
                          }
                        }
                        n132 = Greater?(x=w296, y="Max Exposure - Astrellas") -> (0:w294:bool)
                        n133 = case shown="False" w294 {
                          tunnel: w296 -> [w301 _]
                          frame False {
                            n134 = property on="exposure::13" class="DigNum (strict)"("Val(Sgnl)"=w301) -> ()  [unwired: 2 in, 2 out]
                          }
                          frame True {
                          }
                        }
                      }
                    }
                  }
                  frame #1 {
                    n135 = property on="maxcounts::14" class="DigNum (strict)"() -> ("Value"=w308:dbl)  [unwired: 2 in, 2 out]
                    n136 = Subtract(x="Target - Ghost", y=w308) -> (x-y=w313:dbl)
                    n137 = Absolute Value(x=w313) -> (abs(x)=w311:dbl)
                    n138 = Greater?(x=w311, y="GuardBand Ghost") -> (0:w312:bool)
                    n139 = case shown="True" w312 {
                      tunnel: w313 -> [_ w320]
                      frame False {
                      }
                      frame True {
                        n140 = Greater Than 0?(x=w320) -> (x > 0?=w319:bool)
                        n141 = property on="exposure::14" class="DigNum (strict)"() -> ("Value"=w318:dbl)  [unwired: 2 in, 2 out]
                        n142 = case shown="True" w319 {
                          tunnel: w318 -> [w324 w327]
                          tunnel: "Exposure Step Size - Ghost" -> [w323 w326]
                          tunnel: [w322 w325] -> w314
                          frame False {
                            n143 = Subtract(x=w324, y=w323) -> (x-y=w322:dbl)
                          }
                          frame True {
                            n144 = Add(x=w327, y=w326) -> (x+y=w325:dbl)
                          }
                        }
                        n145 = Greater?(x=w314, y="Max Exposure - Ghost") -> (0:w315:bool)
                        n146 = case shown="False" w315 {
                          tunnel: w314 -> [w321 _]
                          frame False {
                            n147 = property on="exposure::14" class="DigNum (strict)"("Val(Sgnl)"=w321) -> ()  [unwired: 2 in, 2 out]
                          }
                          frame True {
                          }
                        }
                      }
                    }
                  }
                  frame #2 {
                    n148 = property on="maxcounts::15" class="DigNum (strict)"() -> ("Value"=w328:dbl)  [unwired: 2 in, 2 out]
                    n149 = Subtract(x="Target - EC", y=w328) -> (x-y=w333:dbl)
                    n150 = Absolute Value(x=w333) -> (abs(x)=w331:dbl)
                    n151 = Greater?(x=w331, y="GuardBand - EC") -> (0:w332:bool)
                    n152 = case shown="True" w332 {
                      tunnel: w333 -> [_ w340]
                      frame False {
                      }
                      frame True {
                        n153 = Greater Than 0?(x=w340) -> (x > 0?=w339:bool)
                        n154 = property on="exposure::15" class="DigNum (strict)"() -> ("Value"=w334:dbl)  [unwired: 2 in, 2 out]
                        n155 = case shown="True" w339 {
                          tunnel: w334 -> [w344 w347]
                          tunnel: "Exposure Step Size -EC" -> [w343 w346]
                          tunnel: [w342 w345] -> w335
                          frame False {
                            n156 = Subtract(x=w344, y=w343) -> (x-y=w342:dbl)
                          }
                          frame True {
                            n157 = Add(x=w347, y=w346) -> (x+y=w345:dbl)
                          }
                        }
                        n158 = Greater?(x=w335, y="Max Exposure -EC") -> (0:w336:bool)
                        n159 = case shown="False" w336 {
                          tunnel: w335 -> [w341 _]
                          frame False {
                            n160 = property on="exposure::15" class="DigNum (strict)"("Val(Sgnl)"=w341) -> ()  [unwired: 2 in, 2 out]
                          }
                          frame True {
                          }
                        }
                      }
                    }
                  }
                  frame #3 {
                    n161 = property on="maxcounts::16" class="DigNum (strict)"() -> ("Value"=w348:dbl)  [unwired: 2 in, 2 out]
                    n162 = Subtract(x="Target -  NFProfile", y=w348) -> (x-y=w353:dbl)
                    n163 = Absolute Value(x=w353) -> (abs(x)=w351:dbl)
                    n164 = Greater?(x=w351, y="GuardBand - NFProfile") -> (0:w352:bool)
                    n165 = case shown="True" w352 {
                      tunnel: w353 -> [_ w360]
                      frame False {
                      }
                      frame True {
                        n166 = property on="exposure::16" class="DigNum (strict)"() -> ("Value"=w354:dbl)  [unwired: 2 in, 2 out]
                        n167 = Greater Than 0?(x=w360) -> (x > 0?=w359:bool)
                        n168 = case shown="True" w359 {
                          tunnel: w354 -> [w364 w367]
                          tunnel: "Exposure Step Size -NFProfile" -> [w363 w366]
                          tunnel: [w362 w365] -> w355
                          frame False {
                            n169 = Subtract(x=w364, y=w363) -> (x-y=w362:dbl)
                          }
                          frame True {
                            n170 = Add(x=w367, y=w366) -> (x+y=w365:dbl)
                          }
                        }
                        n171 = Greater?(x=w355, y="Max Exposure - NFProfile") -> (0:w356:bool)
                        n172 = case shown="False" w356 {
                          tunnel: w355 -> [w361 _]
                          frame False {
                            n173 = property on="exposure::16" class="DigNum (strict)"("Val(Sgnl)"=w361) -> ()  [unwired: 2 in, 2 out]
                          }
                          frame True {
                          }
                        }
                      }
                    }
                  }
                  frame #4 {
                    n174 = property on="maxcounts::17" class="DigNum (strict)"() -> ("Value"=w368:dbl)  [unwired: 2 in, 2 out]
                    n175 = Subtract(x="Target - SpolGhost", y=w368) -> (x-y=w373:dbl)
                    n176 = Absolute Value(x=w373) -> (abs(x)=w371:dbl)
                    n177 = Greater?(x=w371, y="GuardBand - SpolGhost") -> (0:w372:bool)
                    n178 = case shown="True" w372 {
                      tunnel: w373 -> [_ w380]
                      frame False {
                      }
                      frame True {
                        n179 = property on="exposure::17" class="DigNum (strict)"() -> ("Value"=w374:dbl)  [unwired: 2 in, 2 out]
                        n180 = Greater Than 0?(x=w380) -> (x > 0?=w379:bool)
                        n181 = case shown="True" w379 {
                          tunnel: w374 -> [w384 w387]
                          tunnel: "Exposure Step Size - SpolGhost" -> [w383 w386]
                          tunnel: [w382 w385] -> w375
                          frame False {
                            n182 = Subtract(x=w384, y=w383) -> (x-y=w382:dbl)
                          }
                          frame True {
                            n183 = Add(x=w387, y=w386) -> (x+y=w385:dbl)
                          }
                        }
                        n184 = Greater?(x=w375, y="Max Exposure - SpolGhost") -> (0:w376:bool)
                        n185 = case shown="False" w376 {
                          tunnel: w375 -> [w381 _]
                          frame False {
                            n186 = property on="exposure::17" class="DigNum (strict)"("Val(Sgnl)"=w381) -> ()  [unwired: 2 in, 2 out]
                          }
                          frame True {
                          }
                        }
                      }
                    }
                  }
                  frame #5 {
                    n187 = property on="maxcounts::18" class="DigNum (strict)"() -> ("Value"=w388:dbl)  [unwired: 2 in, 2 out]
                    n188 = Subtract(x="Target -  MantaG", y=w388) -> (x-y=w393:dbl)
                    n189 = Absolute Value(x=w393) -> (abs(x)=w391:dbl)
                    n190 = Greater?(x=w391, y="GuardBand - MantaG") -> (0:w392:bool)
                    n191 = case shown="True" w392 {
                      tunnel: w393 -> [_ w400]
                      frame False {
                      }
                      frame True {
                        n192 = property on="exposure::18" class="DigNum (strict)"() -> ("Value"=w394:dbl)  [unwired: 2 in, 2 out]
                        n193 = Greater Than 0?(x=w400) -> (x > 0?=w399:bool)
                        n194 = case shown="True" w399 {
                          tunnel: w394 -> [w404 w407]
                          tunnel: "Exposure Step Size - MantaG" -> [w403 w406]
                          tunnel: [w402 w405] -> w395
                          frame False {
                            n195 = Subtract(x=w404, y=w403) -> (x-y=w402:dbl)
                          }
                          frame True {
                            n196 = Add(x=w407, y=w406) -> (x+y=w405:dbl)
                          }
                        }
                        n197 = Greater?(x=w395, y="Max Exposure - MantaG") -> (0:w396:bool)
                        n198 = case shown="False" w396 {
                          tunnel: w395 -> [w401 _]
                          frame False {
                            n199 = property on="exposure::18" class="DigNum (strict)"("Val(Sgnl)"=w401) -> ()  [unwired: 2 in, 2 out]
                          }
                          frame True {
                          }
                        }
                      }
                    }
                  }
                  frame #6 {
                    n200 = property on="maxcounts::19" class="DigNum (strict)"() -> ("Value"=w408:dbl)  [unwired: 2 in, 2 out]
                    n201 = Subtract(x="Target -  AstrellaM", y=w408) -> (x-y=w413:dbl)
                    n202 = Absolute Value(x=w413) -> (abs(x)=w411:dbl)
                    n203 = Greater?(x=w411, y="GuardBand - AstrellaM") -> (0:w412:bool)
                    n204 = case shown="True" w412 {
                      tunnel: w413 -> [_ w420]
                      frame False {
                      }
                      frame True {
                        n205 = property on="exposure::19" class="DigNum (strict)"() -> ("Value"=w414:dbl)  [unwired: 2 in, 2 out]
                        n206 = Greater Than 0?(x=w420) -> (x > 0?=w419:bool)
                        n207 = case shown="True" w419 {
                          tunnel: w414 -> [w424 w427]
                          tunnel: "Exposure Step Size - AstrellaM" -> [w423 w426]
                          tunnel: [w422 w425] -> w415
                          frame False {
                            n208 = Subtract(x=w424, y=w423) -> (x-y=w422:dbl)
                          }
                          frame True {
                            n209 = Add(x=w427, y=w426) -> (x+y=w425:dbl)
                          }
                        }
                        n210 = Greater?(x=w415, y="Max Exposure - AstrellaM") -> (0:w416:bool)
                        n211 = case shown="False" w416 {
                          tunnel: w415 -> [w421 _]
                          frame False {
                            n212 = property on="exposure::19" class="DigNum (strict)"("Val(Sgnl)"=w421) -> ()  [unwired: 2 in, 2 out]
                          }
                          frame True {
                          }
                        }
                      }
                    }
                  }
                }
              }
            }
            n213 = local write "timer"(w286) -> ()
          }
        }
        n214 = call <vilib>:"Add State(s) to Queue__jki_lib_state_machine.vi"("State(s) in (\"\")"=w284) -> ("States Out"=w283:string)  [unwired: 14 in]
      }
      frame "Action: Check Mode Wedge" {
        n215 = property on="Position.Axis 3::7" class="DigNum (strict)"() -> ("Value"=w430:dbl)  [unwired: 2 in, 2 out]
        n216 = Subtract(x=w430, y=23.0 ("Position.Axis 3::7")) -> (x-y=w433:dbl)
        n217 = Absolute Value(x=w433) -> (abs(x)=w432:dbl)
        n218 = Less?(x=w432, y=0.05) -> (x < y?=w428:bool)
        n219 = property on="Mode Wedge Button" class="Bool (strict)"("Value"=w428) -> ()  [unwired: 2 in, 2 out]
        n220 = call <vilib>:"Add State(s) to Queue__jki_lib_state_machine.vi"("State(s) in (\"\")"=w437) -> ("States Out"=w436:string)  [unwired: 14 in]
      }
      frame "Action: Check P-Pol Blocker" {
        n221 = property on="pos.Channel0::10" class="Enum (strict)"() -> ("Value"=w440:enum16{"1", "2", "3", "4", "5", "6"})  [unwired: 2 in, 2 out]
        n222 = Equal?(x=w440, y=enum16{"1", "2", "3", "4", "5", "6"}."6" ("pos.Channel0::10")) -> (x = y?=w439:bool)
        n223 = property on="p-pol only button" class="Bool (strict)"("Value"=w439) -> ()  [unwired: 2 in, 2 out]
        n224 = call <vilib>:"Add State(s) to Queue__jki_lib_state_machine.vi"("State(s) in (\"\")"=w444) -> ("States Out"=w443:string)  [unwired: 14 in]
      }
      frame "Action: Update Energy Display" {
        n225 = call "get_laser_energy.vi"("round trip"="value8::1", "HWP angle"="value7::1", "Astrella Power"="Astrella Power") -> ("Attenuated Power"=→"Attenuated  Power":dbl, "HCF output power"=→"HCF output energy":dbl, "FF input energy"=→"FF input calculated":dbl)  [unwired: 6 in]
        n226 = call <vilib>:"Add State(s) to Queue__jki_lib_state_machine.vi"("State(s) in (\"\")"=w454) -> ("States Out"=w453:string)  [unwired: 14 in]
      }
      frame "Action: Update FF Energy" {
        n227 = call "convert_NFProfileOL_count_to_energy.vi"("exposure"="exposure::12", "slope"="value12::1", "mean count"="MeanCounts::12") -> ("energy"=w455:dbl)  [unwired: 8 in]
        "FF Output OL" <- w455
        n228 = call "convert_NFProfileOL_count_to_energy.vi"("exposure"="exposure::16", "slope"="value10::1", "mean count"="MeanCounts::16") -> ("energy"=w460:dbl)  [unwired: 8 in]
        "FF input OL" <- w460
        n229 = Divide(x=w460, y=w455) -> (x/y=w459:dbl)
        n230 = expression code="x*100"(w459) -> (w458:dbl)
        n231 = Bundle("energy"=w460, "energy"=w455, w458) -> (→"chart":cluster{"energy":dbl, "energy":dbl, dbl})  [unwired: 1 in]
        n232 = call <vilib>:"Add State(s) to Queue__jki_lib_state_machine.vi"("State(s) in (\"\")"=w469) -> ("States Out"=w468:string)  [unwired: 14 in]
      }
    }
  }
